vi "incrementRate.vi"(8 "error in (no error)":errorcluster, 11 "Model in":refnum<class "Model.lvclass">) -> (0 "error out":errorcluster, 3 "Model out":refnum<class "Model.lvclass">)   [LabVIEW 2015]
uses:
  Model.lvclass
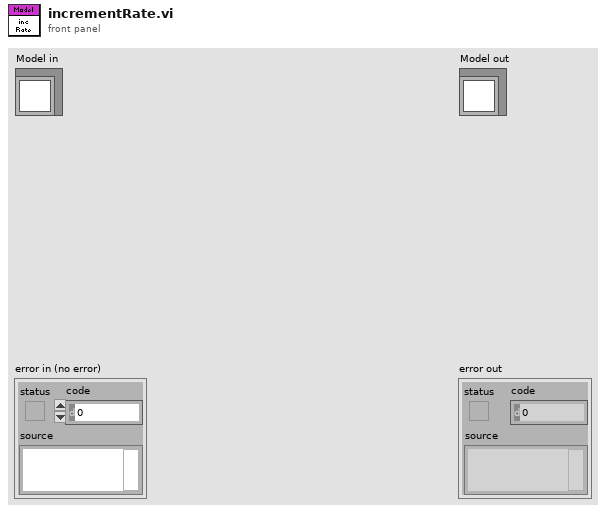
[diagram p1: front panel]
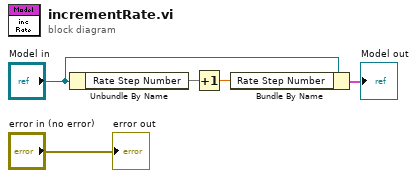
[diagram p0: block diagram]
diagram:
  n1 = Unbundle By Name("Model in") -> ("Rate Step Number"=w3)
  n2 = Increment(x=w3) -> (x+1=w4:dbl)
  n3 = Bundle By Name(cluster="Model in", "Rate Step Number"=w4) -> (→"Model out":cluster{})
  "error out" <- "error in (no error)"
